vi "服务器.vi"() -> ()   [LabVIEW 2017]
uses:
  <vilib>/Analysis/NI_AALBase.lvlib
panel:
  in  "停止":bool
  out "波形图":dbl[](graph)
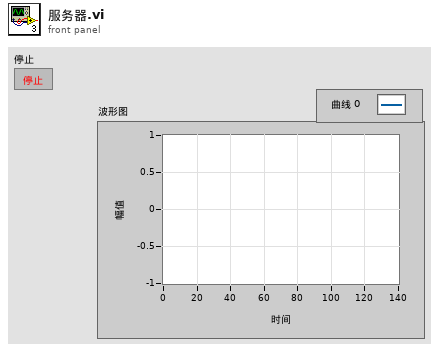
[diagram p1: front panel]
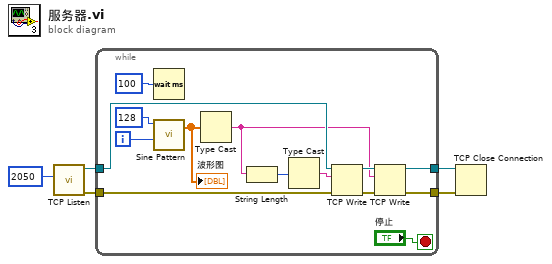
[diagram p0: block diagram]
diagram:
  n1 = call <vilib>:"TCP Listen.vi"("port"=u16 2050) -> ("error out"=w3:errorcluster, "connection ID"=w5:refnum<k5>)  [unwired: 6 in, 3 out]
  n2 = while {
    tunnel: w5 -> [w19]
    tunnel: [w17] -> w4
    tunnel: w3 -> [w16]
    tunnel: [w14] -> w2
    i -> [w12]
    stop <- "停止" stop-if-true
    n3 = Wait (ms)(milliseconds to wait=u32 100 ("等待时间（毫秒）")) -> ()  [unwired: 1 out]
    n4 = call <vilib>:"Sine Pattern.vi"("phase(degrees)"=w12, "samples"=128) -> ("Sinusoidal Pattern"=w8:dbl[])  [unwired: 2 in, 1 out]
    "波形图" <- w8
    n5 = Type Cast(x=w8) -> (*(type *) &x=w9:string)  [unwired: 1 in]
    n6 = String Length(string=w9) -> (length=w11:i32)
    n7 = Type Cast(x=w11) -> (*(type *) &x=w10:string)  [unwired: 1 in]
    n8 = TCP Write(connection ID=w19, data in=w10, error in (no error)=w16) -> (connection ID out=w18:refnum<k5>, error out=w15:errorcluster)  [unwired: 1 in, 1 out]
    n9 = TCP Write(connection ID=w18, data in=w9, error in (no error)=w15) -> (connection ID out=w17:refnum<k5>, error out=w14:errorcluster)  [unwired: 1 in, 1 out]
  }
  n10 = TCP Close Connection(connection ID=w4, error in (no error)=w2) -> ()  [unwired: 1 in, 2 out]
